vi "Config GUI - Add To Project.vi"(8 "error in":errorcluster, 10 "User VI Owner Status":T1, 11 "GUI Objects":T2) -> (0 "error out":errorcluster, 3 "References of In-Memory Projects":refnum<vi>[](array[refnum]))   [LabVIEW 2022 SP3]
doc: "Configures the GUI objects that play a part in the functionality that adds a newly created VI or CTL to an in-memory project."
uses:
  GUI Objects (cluster).ctl
  Owner Status (enum).ctl
  <vilib>/Utility/miscctls.llb/LVFontTypeDef.ctl
panel:
  out "In-Memory Projects":string[](array[string])
  # "Development\ncontrols/indicators useful for development and testing, but which are not outputs of the VI"
  # "Input\nInputs to the VI"
  # "Output\nOutputs of the VI"
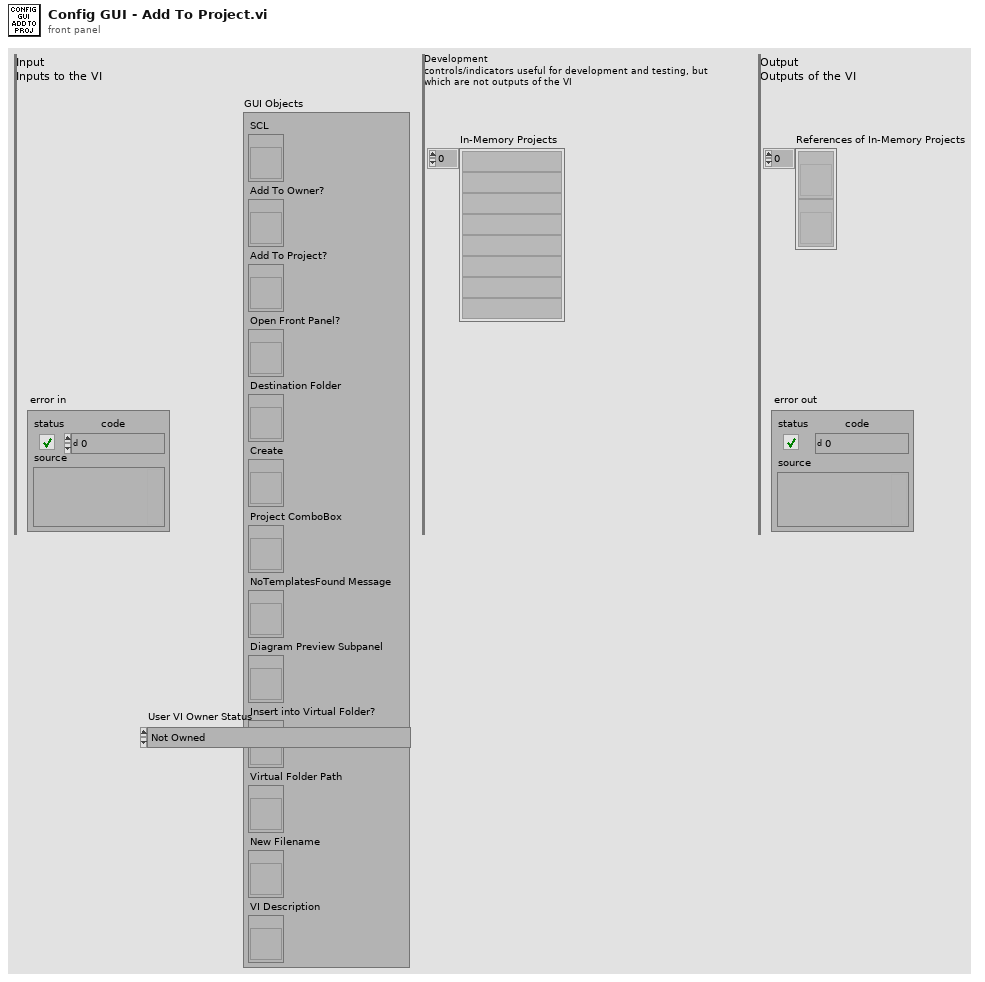
[diagram p1: front panel]
types:
  T1 = typedef "Owner Status (enum).ctl" = enum16{"Not Owned", "Owned by Library (lvlib)", "Owned by Class (lvclass)"}
  T2 = typedef "GUI Objects (cluster).ctl" = cluster{"SCL":refnum<vi>, "Add To Owner?":refnum<vi>, "Add To Project?":refnum<vi>, "Open Front Panel?":refnum<vi>, "Destination Folder":refnum<vi>, "Create":refnum<vi>, "Project ComboBox":refnum<vi>, "NoTemplatesFound Message":refnum<vi>, "Diagram Preview Subpanel":refnum<vi>, "Insert into Virtual Folder?":refnum<vi>, "Virtual Folder Path":refnum<vi>, "New Filename":refnum<vi>, "VI Description":refnum<vi>}
  T3 = typedef "LVFontTypeDef.ctl" = cluster{"Font Name":string, "Size":u16, "Bold":bool, "Italic":bool, "Underline":bool, "Strikeout":bool, "Color":u32}
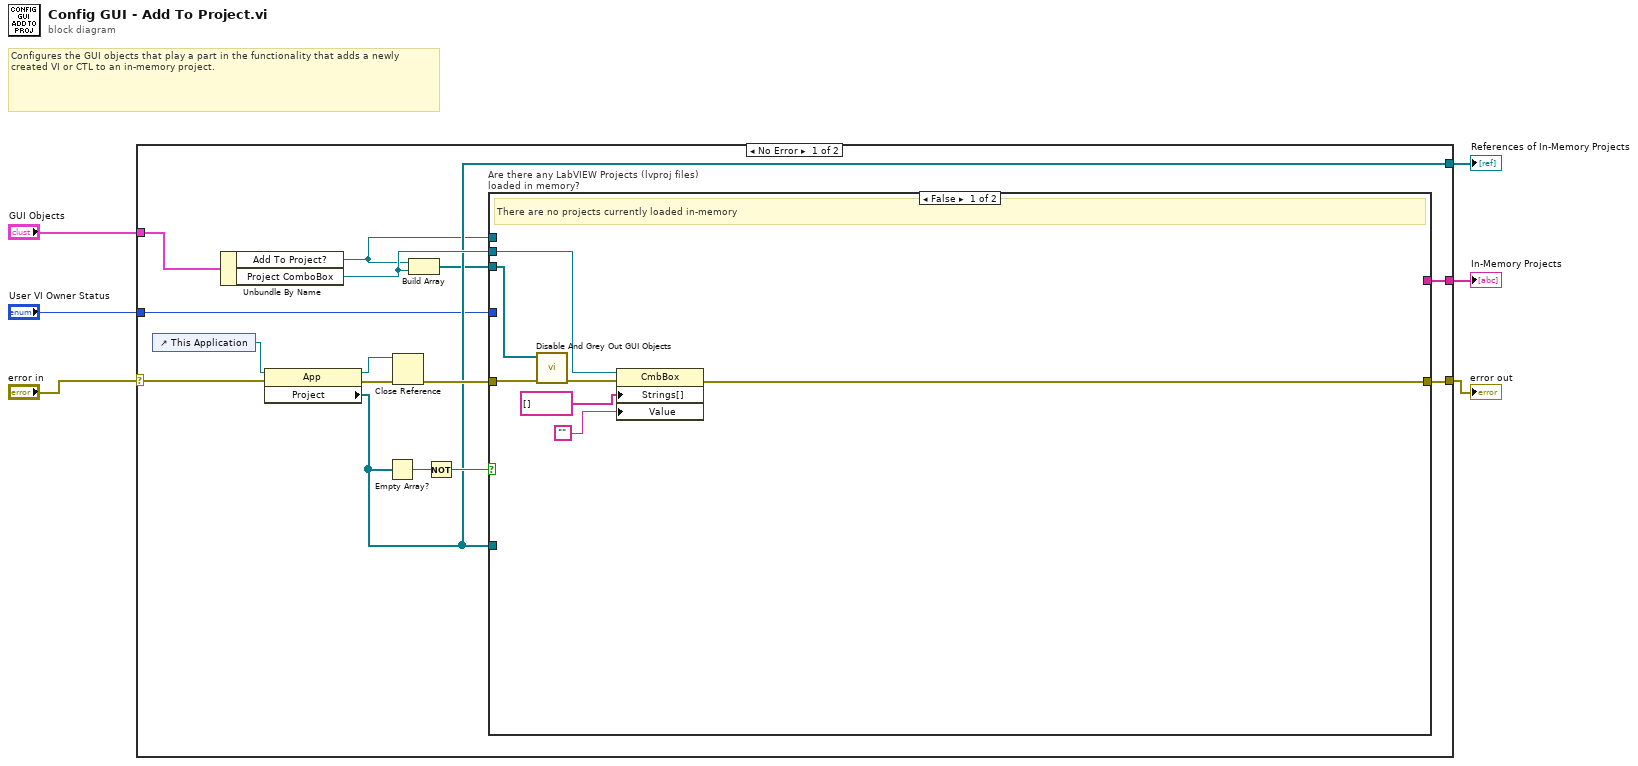
[diagram p0: block diagram]
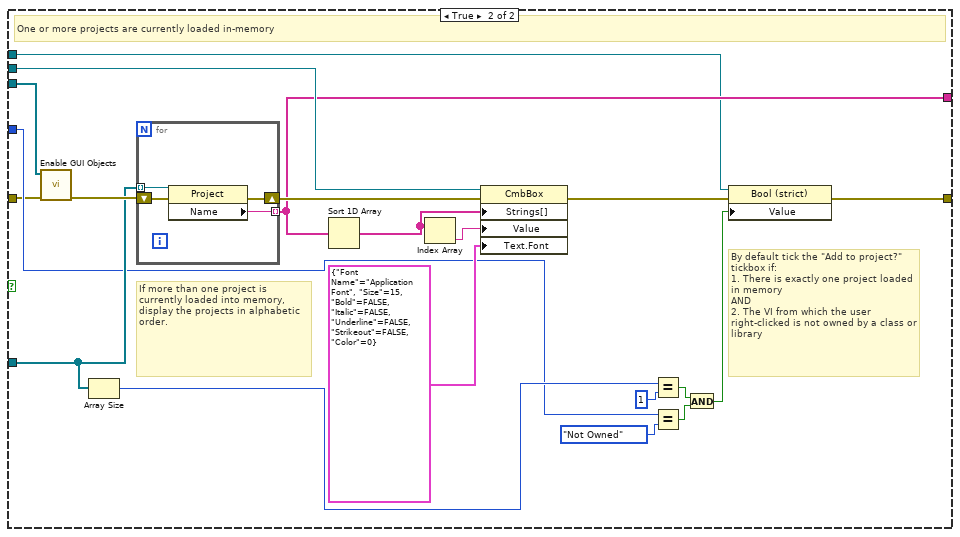
[diagram p2: hidden frame]
diagram:
  # "Configures the GUI objects that play a part in the functionality that adds a newly created VI or CTL to an in-memory project."
  n1 = case shown="No Error" "error in" {
    selector: "error in" -> [w20 w53]
    tunnel: [w14 w53] -> w5
    tunnel: "GUI Objects" -> [w21 _]
    tunnel: [w12 _] -> w3
    tunnel: [w10 _] -> w2
    tunnel: "User VI Owner Status" -> [w8 _]
    frame No Error {
      n2 = control-ref of="This Application"() -> (w18:refnum<vi>)
      n3 = Unbundle By Name(w21) -> ("Add To Project?"=w7:refnum<vi>, "Project ComboBox"=w13:refnum<vi>)
      n4 = property class="App"(reference=w18, error in=w20) -> (reference out=w16:refnum<vi>, error out=w19:errorcluster, "Project"=w10:refnum<vi>[])
      n5 = Empty Array?(array=w10) -> (empty?=w15:bool)
      n6 = Close Reference(reference=w16, error in (no error)=w19) -> (error out=w17:errorcluster)
      n7 = Build Array(w7, w13) -> (w9:refnum<vi>[])
      n8 = Not(x=w15) -> (.not. x?=w11:bool)
      n9 = case "Are there any LabVIEW Projects (lvproj files) loaded in memory?" shown="False" w11 {
        tunnel: w17 -> [w23 w29]
        tunnel: w10 -> [_ w38]
        tunnel: [w27 w40] -> w14
        tunnel: w13 -> [w26 w46]
        tunnel: [_ w43] -> w12
        tunnel: w9 -> [w22 w30]
        tunnel: w8 -> [_ w33]
        tunnel: w7 -> [_ w39]
        frame False {
          # "There are no projects currently loaded in-memory"
          n10 = call "Disable And Grey Out GUI Objects.vi"("Error In"=w23, "GUI Object Refs"=w22) -> ("Error Out"=w28:errorcluster)  [unwired: 9 in]
          n11 = property class="CmbBox"(reference=w26, error in=w28, "Strings[]"=string[] [] ("Strings []"), "Value"="") -> (error out=w27:errorcluster)  [unwired: 1 out]
        }
        frame True {
          # "If more than one project is currently loaded into memory, display the projects in alphabetic order."
          # "By default tick the \"Add to project?\" tickbox if:\n1. There is exactly one project loaded in memory\nAND\n2. The VI from which the user right-clicked is not owned by a class or library"
          # "One or more projects are currently loaded in-memory"
          n12 = call "Enable GUI Objects.vi"("Error In"=w29, "GUI Object Refs"=w30) -> ("Error Out"=w41:errorcluster)  [unwired: 9 in]
          n13 = Array Size(array=w38) -> (size(s)=w37:i32)
          n14 = for {
            shift-right: [w51] -> w48
            shift-left: w41 -> [w52]
            tunnel: w38 -> [w50] mode=indexing
            tunnel: [w49] -> w43 mode=indexing
            n15 = property class="Project"(reference=w50, error in=w52) -> (error out=w51:errorcluster, "Name"=w49:string)  [unwired: 1 out]
          }
          n16 = Sort 1D Array(array=w43) -> (sorted array=w45:string[])
          n17 = Index Array(array=w45) -> (element=w44:string)  [unwired: 1 in]
          n18 = property class="CmbBox"(reference=w46, error in=w48, "Strings[]"=w45, "Value"=w44, "Text.Font"=T3 {"Font Name"="Application Font", "Size"=15, "Bold"=FALSE, "Italic"=FALSE, "Underline"=FALSE, "Strikeout"=FALSE, "Color"=0}) -> (error out=w47:errorcluster)  [unwired: 1 out]
          n19 = Equal?(x=w37, y=1) -> (x = y?=w36:bool)
          n20 = Equal?(x=w33, y=Owner_Status_(enum)."Not Owned") -> (x = y?=w35:bool)
          n21 = And(x=w36, y=w35) -> (x .and. y?=w31:bool)
          n22 = property class="Bool (strict)"(reference=w39, error in=w47, "Value"=w31) -> (error out=w40:errorcluster)  [unwired: 1 out]
        }
      }
    }
    frame Error {
    }
  }
  "error out" <- w5
  "In-Memory Projects" <- w3
  "References of In-Memory Projects" <- w2
